vi "Diagnostic.vi"(2 "Error In":errorcluster) -> (0 "Error Out":errorcluster)   [LabVIEW 2018]
uses:
  Type Defs/Scan Type.ctl
  Type Defs/State Machine.ctl
  Type Defs/GUI Method.ctl
  Type Defs/Lenses.ctl
  GC-MSMSDevlopment/Type/_Mass Range Property.ctl
  GC-MSMSDevlopment/Type/_Mass Range Parameters.ctl
  GC-MSMSDevlopment/Type/_RT Res Type.ctl
  Type Defs/Run Mode.ctl
  Type Defs/Lens Property.ctl
  Type Defs/RT Command.ctl
  <vilib>/Utility/config.llb/Read Key (Path).vi
  <vilib>/Utility/config.llb/NI_LVConfig.lvlib
panel:
  in  "Test PIC":bool
  in  "Lens Value":u32
  out "DAC Value":dbl
  in  "In User Units":bool
  in  "Scan Type":T1
  out "ItemTag":string
  in  "Run":bool
  in  "Lens Table":i32(listbox)
  in  "Method Path":path
  out "Spectrum":dbl[](graph)
  in  "stop":bool
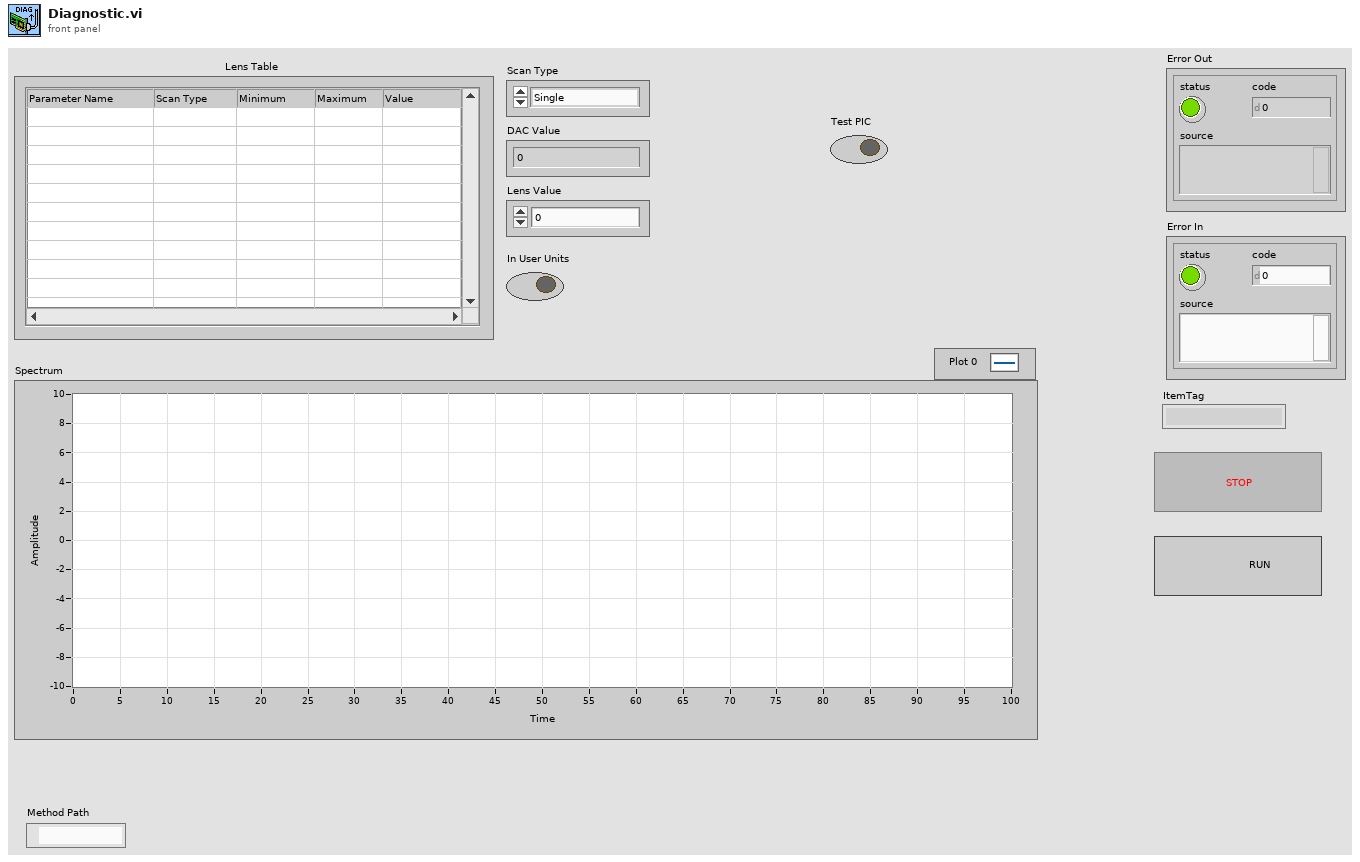
[diagram p1: front panel]
types:
  T1 = typedef "Scan Type.ctl" = enum8{"Single", "Dual", "Ramp"}
  T2 = typedef "GUI Method.ctl" = cluster{"Lenses":T3[], "Mass Ranges":T4[], "Acquire":bool, "MCA":bool, "Q1DC EN":bool, "Q1 POL":bool, "Q3 POL":bool, "Q1 RF  EN":bool, "Averaging":bool, "Log Scale":bool, "CPS":bool, "Units":bool, "Data Path":path, "Run Mode":T7, "Fixed Mass (amu)":dbl, "Q3DC EN":bool, "Q3 RF  EN":bool, "Negative":bool}
  T3 = typedef "Lenses.ctl" = cluster{"Scan Type":u8, "Scans":i32, "Time 1":dbl, "Time 2":dbl, "Value 1":dbl, "Value 2":dbl, "Step Size":dbl}
  T4 = typedef "_Mass Range Property.ctl" = cluster{"Start":dbl, "Stop":dbl, "Step Size":dbl, "Steps":i32, "Dwell":dbl, "Parameters":T5[], "Res":T6}
  T5 = typedef "_Mass Range Parameters.ctl" = cluster{"Name":string, "Ch#":u8, "StartV":dbl, "StopV":dbl, "StepV":dbl, "Index":u8}
  T6 = typedef "_RT Res Type.ctl" = u16
  T7 = typedef "Run Mode.ctl" = enum16{"MRM (Q1/Q2)", "Q1 Scan", "Q1 SRM", "Q2 Scan", "Q2 SRM", "Product Scan", "Precursor Scan", "Neutral Loss", "Neutral Gain"}
  T8 = typedef "State Machine.ctl" = enum16{"Case 0", "Case 1", "Case 2", "Case 3", "Case 4", "Case 5", "Case 6", "Case 7", "Case 8", "Case 9", "Case 10", "Error", "Exit"}
  T9 = cluster{"GUI Methode":T2, "Update":bool, "Running":bool, "Method Path":path}
  T10 = enum16{"open", "replace", "create", "open or create", "replace or create", "replace or create with confirmation"}
  T11 = typedef "Lens Property.ctl" = cluster{"Unit":bool, "Start ":dbl, "Stop ":dbl, "Dwell Time":dbl, "Pause Time":dbl, "Scans":i32, "Step Size":dbl, "Row Numer":i32, "Ramp Time (ms)":i32, "Start DAC":i32, "Scan Type":T1}
  T12 = typedef "RT Command.ctl" = enum16{"xml Start Run", "xml Start Actual Run", "xml Stop Run", "xml Runtime Update", "xml Get Status", "xml Get Table", "xml Set Table", "xml Get Configuration", "xml System Status", "xml Set LC Input Logic", "xml Get Data", "xml Get Info", "Start", "StartActualRun", "Stop", "Runtime Update", "Get Data", "Get Info", "Get Status", "Get Param", "Get Config", "Get Table", "Read ADC", "Set Oscillator", "Update Config", "Update Table", "Set All Pol", "Set Pol and DC", "Set Max Mass", "Toggle RP", "Toggle EL", "Set PIC", "Initialize Turbo", "Send Turbo Comm", "Close Turbo", "P1", "P2", "P3", "Send Serial", "Set LC Out", "Get LC In", "Read VAC", "Test Table", "Toggle Power", "Get Startup", "Set Startup", "Get ADC Table", "Set ADC Table", "Get Brief Status", "Get Detail Status", "Auxiliary Update", "Set CC Logics", "Set CC Input Logics", "Ignore Error", "invalid"}
  T13 = typedef "NI_LVConfig.lvlib/Config Data RefNum.ctl" = refnum<k1>
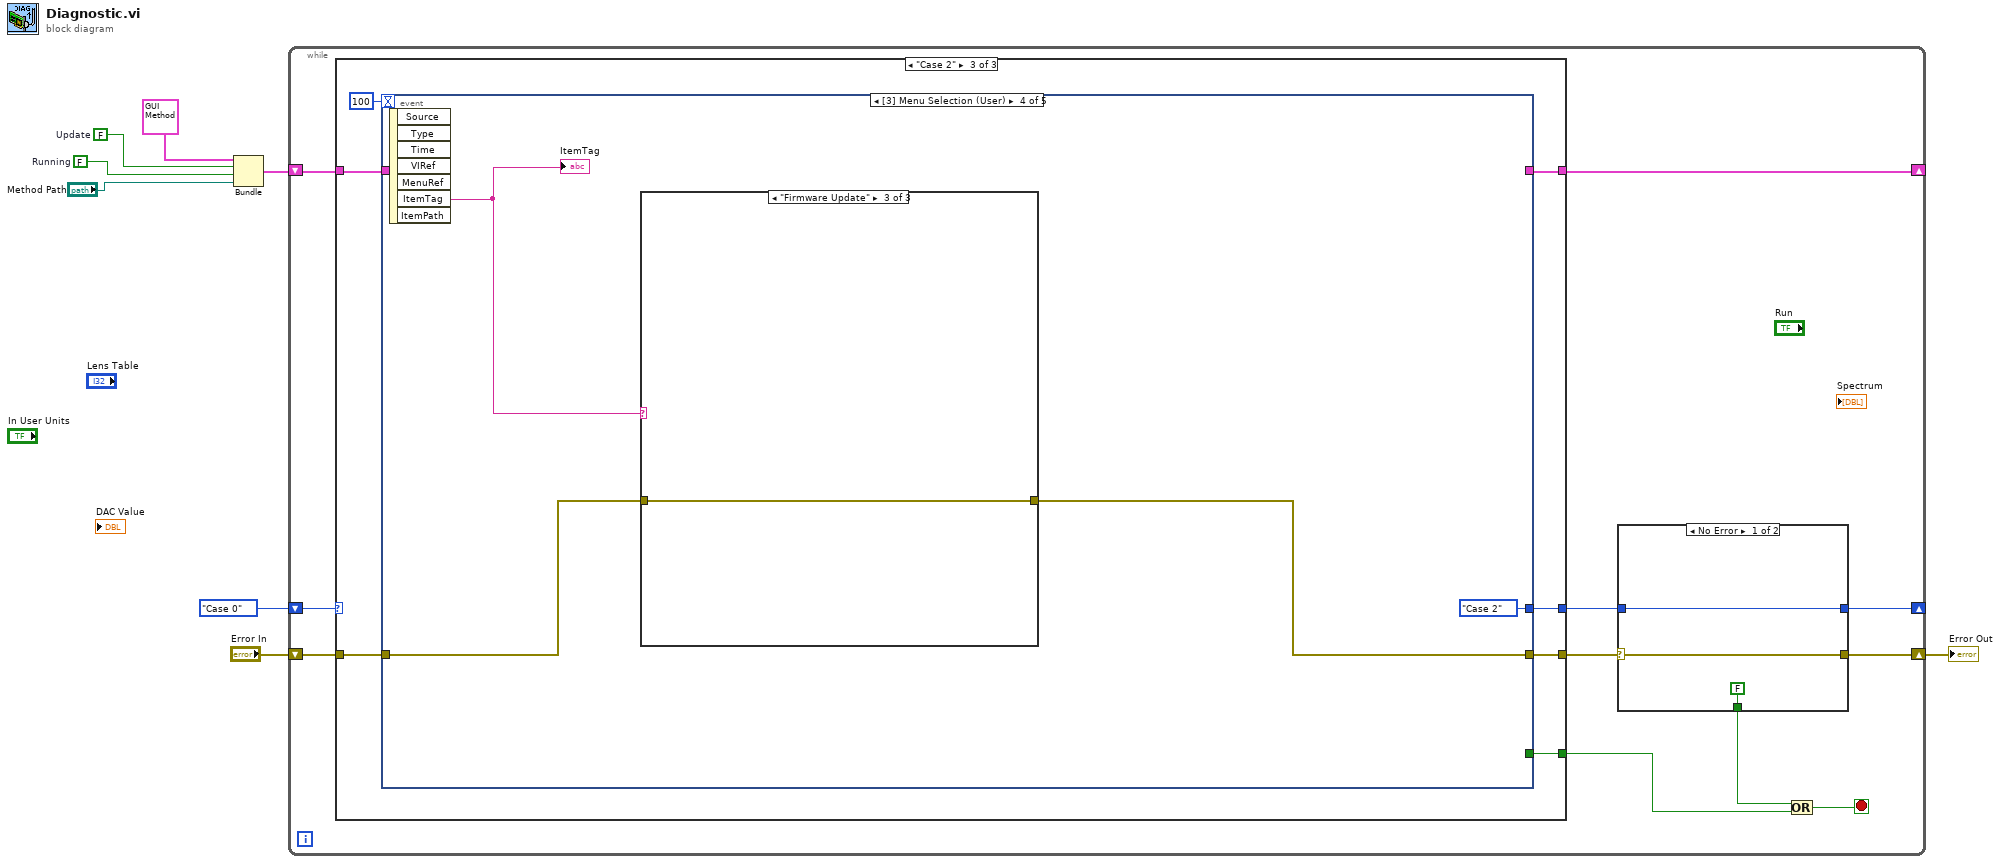
[diagram p0: block diagram]
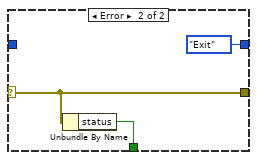
[diagram p2: hidden frame]
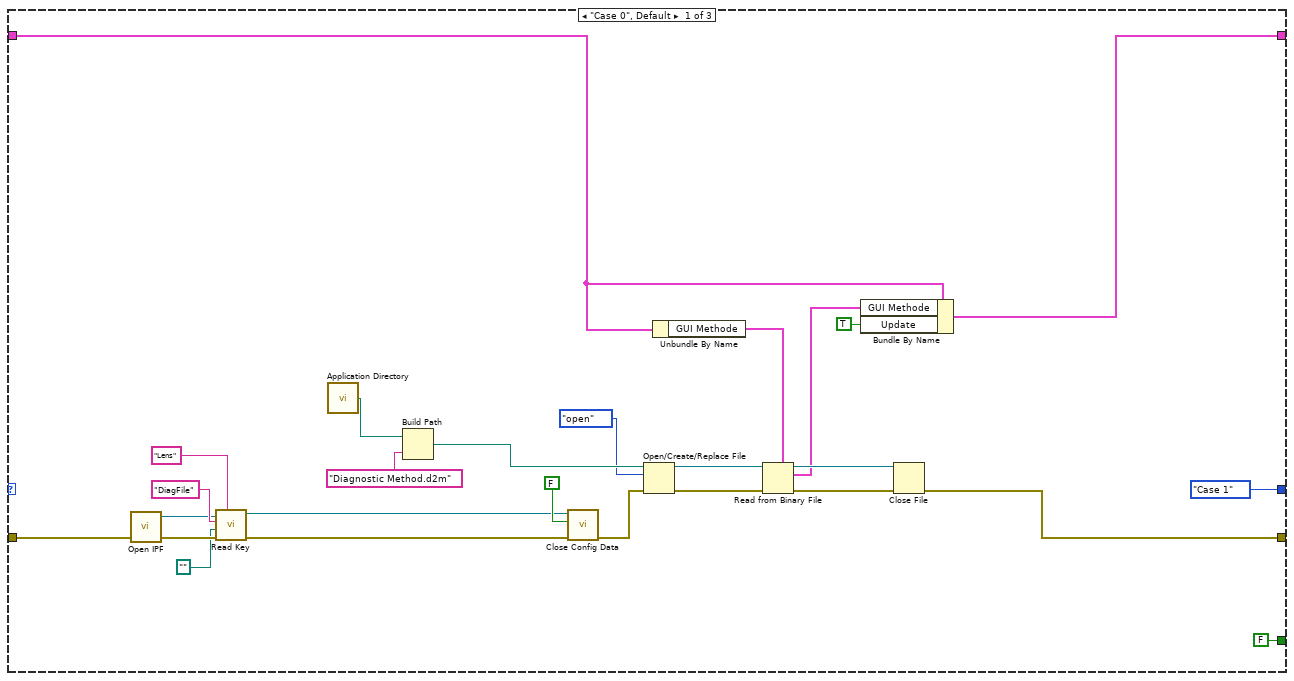
[diagram p3: hidden frame]
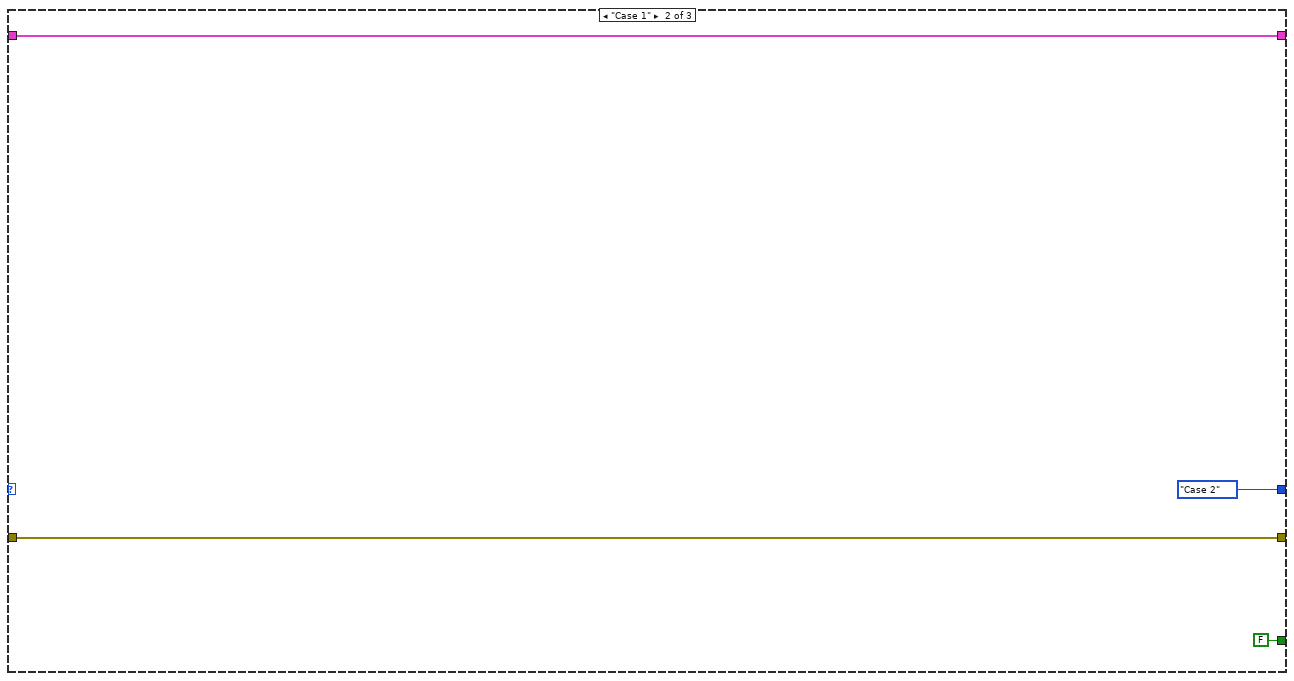
[diagram p4: hidden frame]
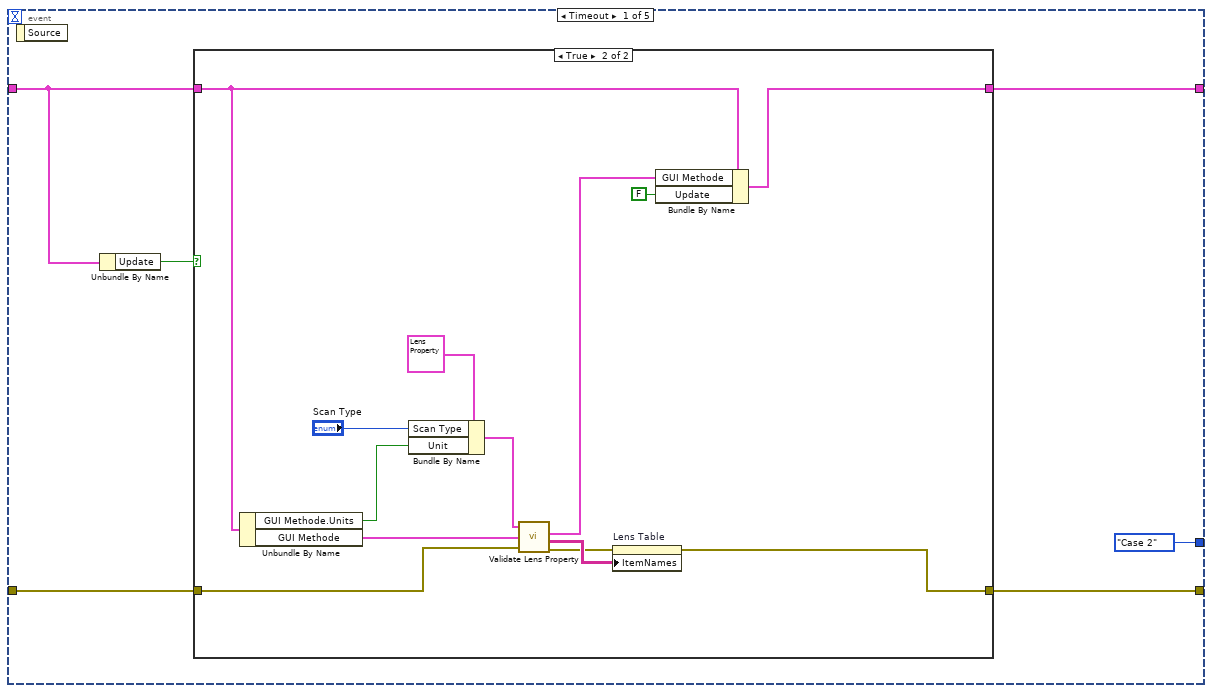
[diagram p5: hidden frame]
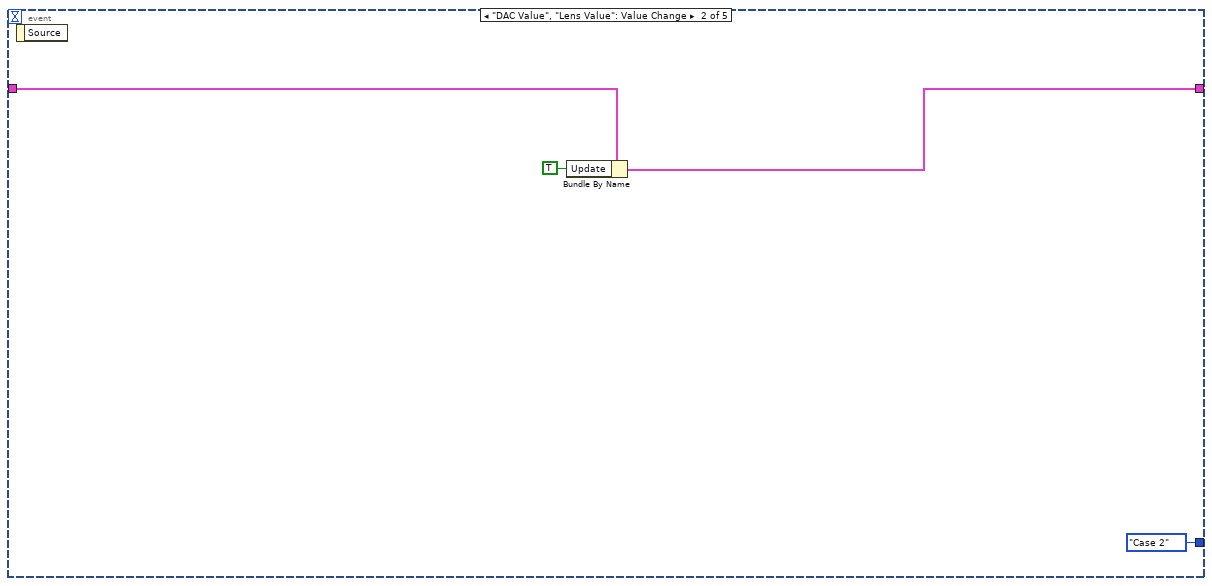
[diagram p7: hidden frame]
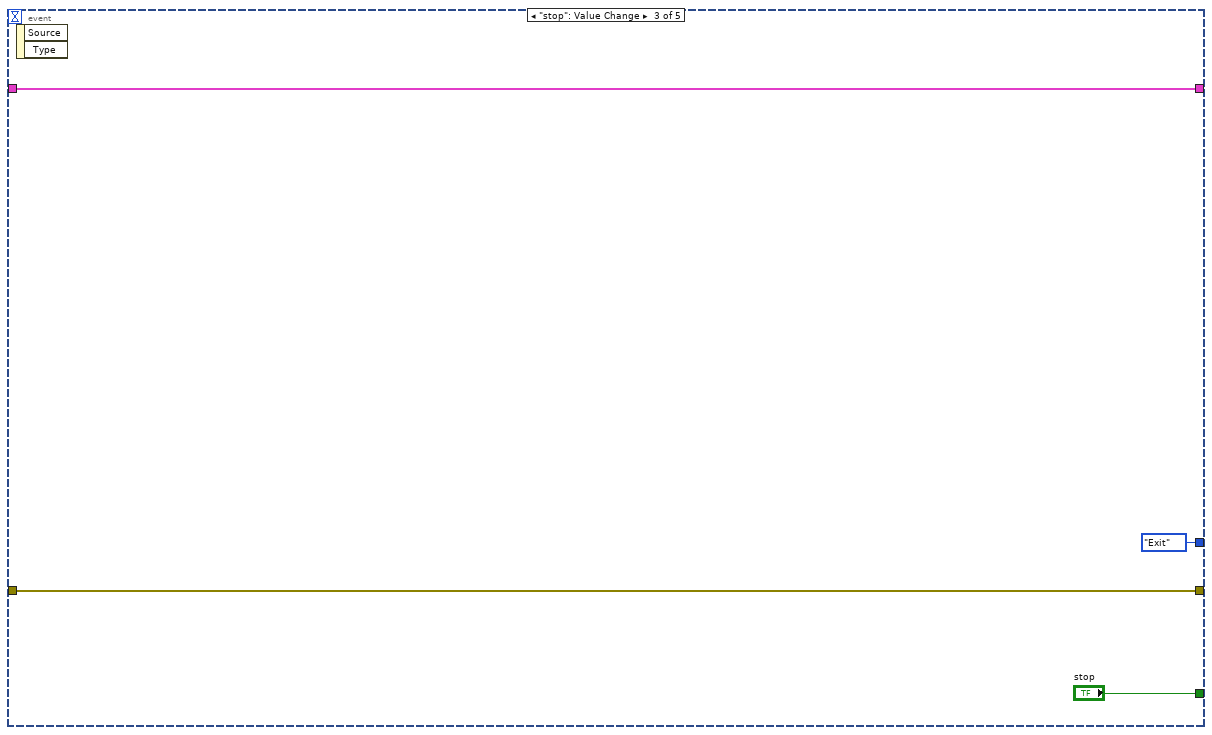
[diagram p8: hidden frame]
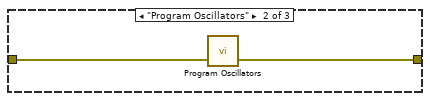
[diagram p10: hidden frame]
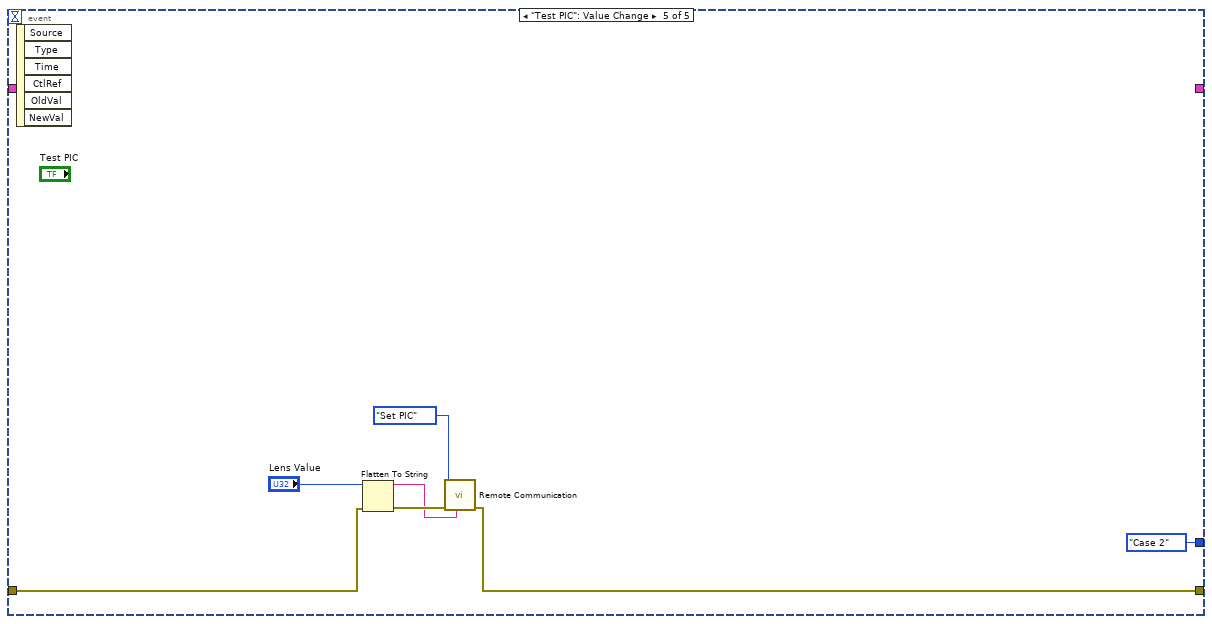
[diagram p11: hidden frame]
diagram:
  w4 = FALSE  # Update
  w3 = FALSE  # Running
  n1 = Bundle("GUI Methode"=T2 {"Lenses"=[], "Mass Ranges"=[], "Acquire"=FALSE, "MCA"=FALSE, "Q1DC EN"=FALSE, "Q1 POL"=FALSE, "Q3 POL"=FALSE, "Q1 RF  EN"=FALSE, "Averaging"=FALSE, "Log Scale"=FALSE, "CPS"=FALSE, "Units"=FALSE, "Data Path"=path "", "Run Mode"=enum."MRM (Q1/Q2)", "Fixed Mass (amu)"=1.0, "Q3DC EN"=FALSE, "Q3 RF  EN"=FALSE, "Negative"=FALSE}, "Update"=w4, "Running"=w3, "Method Path"="Method Path") -> (w1:T9)  [unwired: 1 in]
  n2 = while {
    shift-right: [w18] -> w7
    shift-left: "Error In" -> [w17]
    shift-right: [w13] -> _
    shift-left: State_Machine."Case 0" ("Enum") -> [w19]
    shift-right: [w10] -> _
    shift-left: w1 -> [w11]
    stop <- w16 stop-if-true
    n3 = case shown="\"Case 2\"" w19 {
      tunnel: w17 -> [w50 w53 w58]
      tunnel: [State_Machine."Case 1" ("Enum") State_Machine."Case 2" ("Enum") w59] -> w14
      tunnel: [w37 w53 w57] -> w12
      tunnel: w11 -> [w36 w54 w61]
      tunnel: [w34 w54 w60] -> w10
      tunnel: [FALSE ("stop") FALSE ("stop") w56] -> w9
      frame "Case 0", Default {
        n4 = call "Open IPF.vi"("Error In"=w50) -> ("Error Out"=w49:errorcluster, "IPF refnum"=w45:T13)  [unwired: 2 in, 1 out]
        n5 = call-poly <vilib>:"Read Key.vi"("section"="Lens", "error in (no error)"=w49, "default value"=path "", "key"="DiagFile", "refnum"=w45) -> ("error out"=w28:errorcluster, "refnum out"=w43:T13)  [unwired: 5 out]
        n6 = call <vilib>:"Application Directory.vi"() -> ("Application Directory"=w26:path)
        n7 = Build Path(base path=w26, name or relative path="Diagnostic Method.d2m") -> (appended path=w29:path)
        n8 = call <vilib>:"Close Config Data.vi"("error in (no error)"=w28, "write file if changed (T)"=FALSE, "refnum"=w43) -> ("error out"=w42:errorcluster)  [unwired: 7 in, 1 out]
        n9 = Open/Create/Replace File(file path (use dialog)=w29, error in=w42, operation (0:open)=T10."open") -> (refnum out=w40:refnum<file>, error out=w41:errorcluster)  [unwired: 3 in, 1 out]
        n10 = Unbundle By Name(w36) -> ("GUI Methode"=w32:T2)
        n11 = Read from Binary File(5:w32, 8:w41, 11:w40) -> (0:w39:errorcluster, 2:w35:T2, 3:w38:refnum<file>)  [unwired: 3 in, 1 out]
        n12 = Bundle By Name(cluster=w36, "GUI Methode"=w35, "Update"=TRUE) -> (w34:T9)
        n13 = Close File(refnum=w38, error in=w39) -> (error out=w37:errorcluster)  [unwired: 1 out]
      }
      frame "Case 1" {
      }
      frame "Case 2" {
        n14 = event shown="[3] Menu Selection (User)" {
          selector: _ -> [_ _ _ _ _]
          dyn-events: _ -> [_ _ _ _ _]
          timeout: 100 -> [_ _ _ _ _]
          tunnel: w61 -> [w67 w87 w89 _ _]
          tunnel: [w63 w86 w89 _ _] -> w60
          tunnel: [State_Machine."Case 2" ("Enum") State_Machine."Case 2" ("Enum") State_Machine."Exit" ("Enum") State_Machine."Case 2" ("Enum") State_Machine."Case 2" ("Enum")] -> w59
          tunnel: w58 -> [w65 _ w90 w93 w104]
          tunnel: [w64 _ w90 w92 w101] -> w57
          tunnel: [_ _ "stop" _ _] -> w56
          event Timeout {
            n15 = event-data() -> ()  [unwired: 1 in, 1 out]
            n16 = Unbundle By Name(w67) -> ("Update"=w68:bool)
            n17 = case shown="True" w68 {
              tunnel: w67 -> [w69 w78]
              tunnel: [w69 w75] -> w63
              tunnel: w65 -> [w70 w83]
              tunnel: [w70 w80] -> w64
              frame False {
              }
              frame True {
                n18 = Unbundle By Name(w78) -> ("GUI Methode.Units"=w71:bool, "GUI Methode"=w79:T2)
                n19 = Bundle By Name(cluster=T11 {"Unit"=TRUE, "Start "=1.0, "Stop "=1.0, "Dwell Time"=1.0, "Pause Time"=1.0, "Scans"=1, "Step Size"=1.0, "Row Numer"=0, "Ramp Time (ms)"=1, "Start DAC"=0, "Scan Type"=enum."Single"} ("Lens Property"), "Scan Type"="Scan Type", "Unit"=w71) -> (w73:T11)
                n20 = call "Validate Lens Property.vi"("Lens Property In"=w73, "GUI Methode In"=w79, "Error In"=w83) -> ("GUI Methode Out"=w77:T2, "Lens Table"=w82:string[][], "Error Out"=w81:errorcluster)  [unwired: 1 out]
                n21 = property on="Lens Table" class="MCListbox (strict)"(error in=w81, "ItemNames"=w82) -> (error out=w80:errorcluster)  [unwired: 1 in, 1 out]
                n22 = Bundle By Name(cluster=w78, "GUI Methode"=w77, "Update"=FALSE) -> (w75:T9)
              }
            }
          }
          event "DAC Value", "Lens Value": Value Change {
            n23 = event-data() -> ()  [unwired: 1 in, 1 out]
            n24 = Bundle By Name(cluster=w87, "Update"=TRUE) -> (w86:T9)
          }
          event "stop": Value Change {
            n25 = event-data() -> ()  [unwired: 1 in, 2 out]
          }
          event Menu Selection (User) {
            n26 = event-data() -> ("ItemTag"=w94:string)  [unwired: 1 in, 6 out]
            "ItemTag" <- w94
            n27 = case shown="\"Firmware Update\"" w94 {
              tunnel: w93 -> [w96 w98 w99]
              tunnel: [w96 w97 w99] -> w92
              frame "False", Default {
              }
              frame "Program Oscillators" {
                n28 = call "Program Oscillators.vi"("Error In"=w98) -> ("Error Out"=w97:errorcluster)  [unwired: 2 in]
              }
              frame "Firmware Update" {
              }
            }
          }
          event "Test PIC": Value Change {
            n29 = event-data() -> ()  [unwired: 1 in, 6 out]
            n30 = Flatten To String(anything="Lens Value", error in (no error)=w104) -> (data string=w103:string, error out=w106:errorcluster)  [unwired: 3 out]
            n31 = call "Remote Communication.vi"("String"=w103, "Error In"=w106, "Command"=RT_Command."Set PIC") -> ("Error Out"=w101:errorcluster)  [unwired: 3 in, 3 out]
          }
        }
      }
    }
    n32 = case shown="No Error" w12 {
      selector: w12 -> [w22 w24]
      tunnel: [w22 w24] -> w18
      tunnel: [FALSE ("status") w25] -> w15
      tunnel: [w20 State_Machine."Exit" ("Enum")] -> w13
      tunnel: w14 -> [w20 _]
      frame No Error {
      }
      frame Error {
        n33 = Unbundle By Name(w24) -> ("status"=w25:bool)
      }
    }
    n34 = Or(x=w15, y=w9) -> (x .or. y?=w16:bool)
  }
  "Error Out" <- w7
